vi "G#Object_CleanUp.vi"(1 "full class name (\"\")":string, 5 "error in (no error)":errorcluster) -> (15 "any dead objects?":bool, 19 "error out":errorcluster)   [LabVIEW 2017, in "G#Object.lvclass"]
doc: "Cleans up the specified class and remove all \"dead\" object. \"Dead\" object could occur if LabVIEW garbage collector removes objects because the object creating top-level VI stops executing."
uses:
  G#Object.lvclass
  G#Object.lvclass/G#Object.ctl
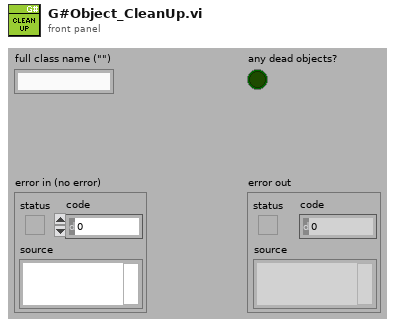
[diagram p1: front panel]
types:
  T1 = cluster{"full class name (\"\")":string, "Ref":refnum<class "G#Object.lvclass">}
  T2 = cluster{"full class name (\"\")":string, "Ref":refnum<class "G#Object.lvclass">}[]
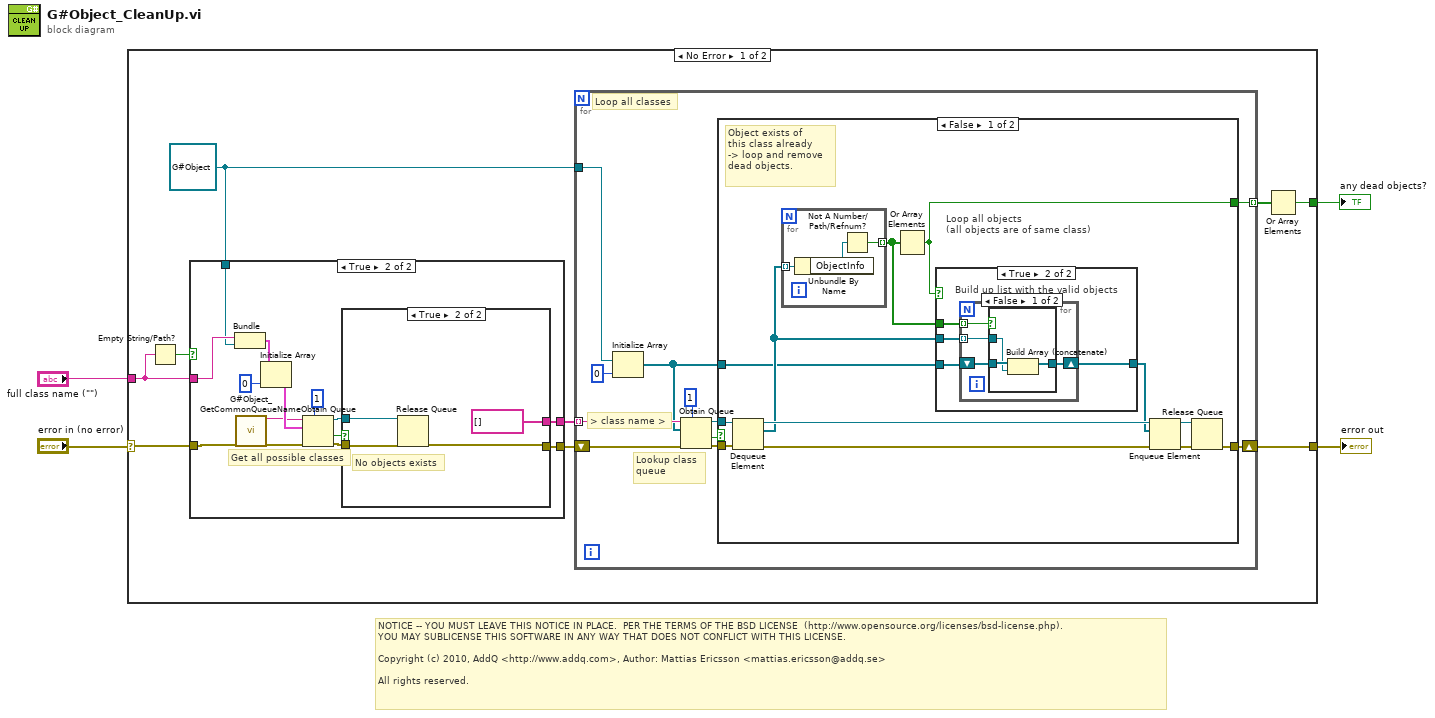
[diagram p0: block diagram]
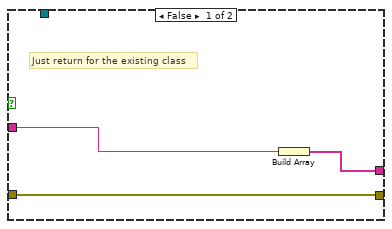
[diagram p2: hidden frame]
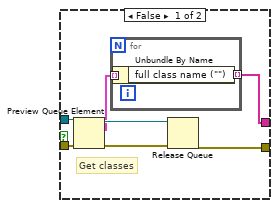
[diagram p3: hidden frame]
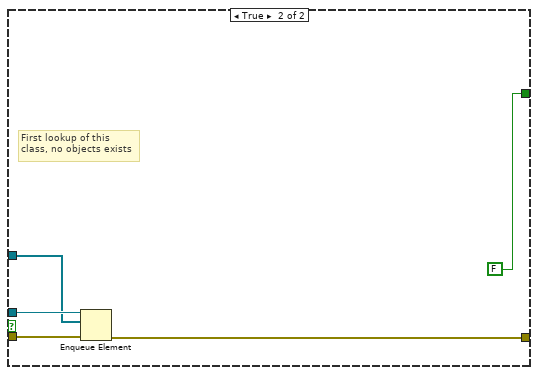
[diagram p6: hidden frame]
diagram:
  # "NOTICE -- YOU MUST LEAVE THIS NOTICE IN PLACE.  PER THE TERMS OF THE BSD LICENSE  (http://www.opensource.org/licenses/bsd-license.php).\nYOU MAY SUBLICENSE THIS SOFTWARE IN ANY WAY THAT DOES NOT CONFLICT WITH THIS LICENSE.\n\nCopyright (c) 2010, AddQ <http://www.addq.com>, Author: Mattias Ericsson <mattias.ericsson@addq.se>\n\nAll rights reserved."
  n1 = case shown="No Error" "error in (no error)" {
    selector: "error in (no error)" -> [w11 w88]
    tunnel: [w10 w88] -> w3
    tunnel: "full class name (\"\")" -> [w8 _]
    tunnel: [w5 _] -> w1
    frame No Error {
      w7 = refnum<class "G#Object.lvclass"> refnum ("Ref")
      n2 = Empty String/Path?(string/path=w8) -> (empty?=w9:bool)
      n3 = case shown="True" w9 {
        tunnel: [w15 w24] -> w13
        tunnel: [w16 w23] -> w12
        tunnel: w11 -> [w16 w19]
        tunnel: w8 -> [w14 w21]
        tunnel: w7 -> [_ w20]
        frame False {
          # "Just return for the existing class"
          n4 = Build Array(w14) -> (w15:string[])
        }
        frame True {
          # "Get all possible classes"
          n5 = Bundle("full class name (\"\")"=w21, "Ref"=w20) -> (w22:T1)  [unwired: 1 in]
          n6 = call "G#Object_GetCommonQueueName.vi"("error in (no error)"=w19) -> ("queue name"=w17:string, "error out"=w18:errorcluster)  [unwired: 17 in]
          n7 = Initialize Array(w22, 0 ("dimension size")) -> (w25:T2)
          n8 = Obtain Queue(max queue size (-1, unlimited)=1, name (unnamed)=w17, element data type=w25, error in (no error)=w18) -> (queue out=w28:refnum<queue>, created new?=w30:bool, error out=w29:errorcluster)  [unwired: 1 in]
          n9 = case shown="True" w30 {
            tunnel: w29 -> [w37 w40]
            tunnel: w28 -> [w36 w41]
            tunnel: [w32 string[] []] -> w24
            tunnel: [w35 w43] -> w23
            frame False {
              # "Get classes"
              n10 = Preview Queue Element(queue=w36, error in (no error)=w37) -> (queue out=w33:refnum<queue>, element=w31:T2, error out=w34:errorcluster)  [unwired: 1 in, 1 out]
              n11 = for {
                tunnel: [w39] -> w32 mode=indexing
                tunnel: w31 -> [w38] mode=indexing
                n12 = Unbundle By Name(w38) -> ("full class name (\"\")"=w39:string)
              }
              n13 = Release Queue(queue=w33, error in (no error)=w34) -> (error out=w35:errorcluster)  [unwired: 1 in, 2 out]
            }
            frame True {
              # "No objects exists"
              n14 = Release Queue(queue=w41, error in (no error)=w40) -> (error out=w43:errorcluster)  [unwired: 1 in, 2 out]
            }
          }
        }
      }
      n15 = for {
        shift-right: [w45] -> w10
        shift-left: w12 -> [w50]
        tunnel: w13 -> [w49] mode=indexing
        tunnel: w7 -> [w46]
        tunnel: [w44] -> w6 mode=indexing
        # "Loop all classes"
        # "> class name >"
        # "Lookup class\nqueue"
        n16 = Initialize Array(w46, 0 ("dimension size")) -> (w48:refnum<class "G#Object.lvclass">[])
        n17 = Obtain Queue(max queue size (-1, unlimited)=1, name (unnamed)=w49, element data type=w48, error in (no error)=w50) -> (queue out=w51:refnum<queue>, created new?=w52:bool, error out=w53:errorcluster)  [unwired: 1 in]
        n18 = case shown="False" w52 {
          tunnel: w53 -> [w65 w87]
          tunnel: w51 -> [w64 w85]
          tunnel: w48 -> [w55 w84]
          tunnel: [w66 w86] -> w45
          tunnel: [w59 FALSE] -> w44
          frame False {
            # "Loop all objects\n(all objects are of same class)"
            # "Object exists of\nthis class already\n-> loop and remove\ndead objects."
            n19 = Dequeue Element(queue=w64, error in (no error)=w65) -> (queue out=w62:refnum<queue>, element=w58:refnum<class "G#Object.lvclass">[], error out=w63:errorcluster)  [unwired: 1 in, 1 out]
            n20 = for {
              tunnel: w58 -> [w81] mode=indexing
              tunnel: [w80] -> w56 mode=indexing
              n21 = Unbundle By Name(w81) -> ("ObjectInfo"=w82:refnum<queue>)
              n22 = Not A Number/Path/Refnum?(number/path/refnum=w82) -> (NaN/Path/Refnum?=w80:bool)
            }
            n23 = Or Array Elements(Boolean array=w56) -> (logical OR=w59:bool)
            n24 = case shown="True" w59 {
              tunnel: w58 -> [w67 w70]
              tunnel: [w67 w68] -> w57
              tunnel: w56 -> [_ w71]
              tunnel: w55 -> [_ w69]
              frame False {
              }
              frame True {
                # "Build up list with the valid objects"
                n25 = for {
                  shift-right: [w73] -> w68
                  shift-left: w69 -> [w74]
                  tunnel: w71 -> [w75] mode=indexing
                  tunnel: w70 -> [w72] mode=indexing
                  n26 = case shown="False" w75 {
                    tunnel: w74 -> [w77 w79]
                    tunnel: [w78 w79] -> w73
                    tunnel: w72 -> [w76 _]
                    frame False {
                      n27 = Build Array (concatenate)(w77, w76) -> (w78:refnum<class "G#Object.lvclass">[])
                    }
                    frame True {
                    }
                  }
                }
              }
            }
            n28 = Enqueue Element(queue=w62, element=w57, error in (no error)=w63) -> (queue out=w60:refnum<queue>, error out=w61:errorcluster)  [unwired: 1 in, 1 out]
            n29 = Release Queue(queue=w60, error in (no error)=w61) -> (error out=w66:errorcluster)  [unwired: 1 in, 2 out]
          }
          frame True {
            # "First lookup of this\nclass, no objects exists"
            n30 = Enqueue Element(queue=w85, element=w84, error in (no error)=w87) -> (error out=w86:errorcluster)  [unwired: 1 in, 2 out]
          }
        }
      }
      n31 = Or Array Elements(Boolean array=w6) -> (logical OR=w5:bool)
    }
    frame Error {
    }
  }
  "error out" <- w3
  "any dead objects?" <- w1
